vi "Framework Main.vi"(8 "error in (no error)":errorcluster, 11 "Framework in":refnum<class "Framework.lvclass">) -> (0 "error out":errorcluster, 3 "Framework out":refnum<class "Framework.lvclass">)   [LabVIEW 2017]
uses:
  Builds/Data Sharing Framework/Current/Data Sharing Framework Core/DSF Core.lvlibp/Engine/Classes/Framework/Framework.lvclass
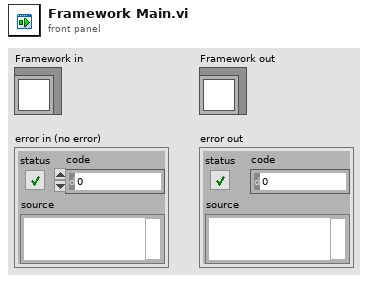
[diagram p1: front panel]
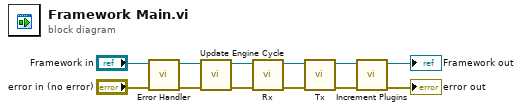
[diagram p0: block diagram]
diagram:
  n1 = call "Error Handler.vi"("error in (no error)"="error in (no error)", "Framework in"="Framework in") -> ("error out"=w12:errorcluster, "Framework out"=w11:refnum<class "Framework.lvclass">)  [unwired: 8 in]
  n2 = call-dynamic "Update Engine Cycle.vi"("error in (no error)"=w12, "Framework in"=w11) -> ("error out"=w2:errorcluster, "Framework out"=w1:refnum<class "Framework.lvclass">)  [unwired: 8 in]
  n3 = call "Rx.vi"("error in (no error)"=w2, "Framework in"=w1) -> ("error out"=w4:errorcluster, "Framework out"=w3:refnum<class "Framework.lvclass">)  [unwired: 8 in]
  n4 = call "Tx.vi"("error in (no error)"=w4, "Framework in"=w3) -> ("error out"=w5:errorcluster, "Framework out"=w6:refnum<class "Framework.lvclass">)  [unwired: 8 in]
  n5 = call "Increment Plugins.vi"("error in (no error)"=w5, "Framework in"=w6) -> ("error out"=→"error out":errorcluster, "Framework out"=→"Framework out":refnum<class "Framework.lvclass">)  [unwired: 8 in]
